vi "PhidgetClose.vi"(8 "error in":errorcluster, 11 "Device In":i32) -> (0 "error out":errorcluster)   [LabVIEW 2013]
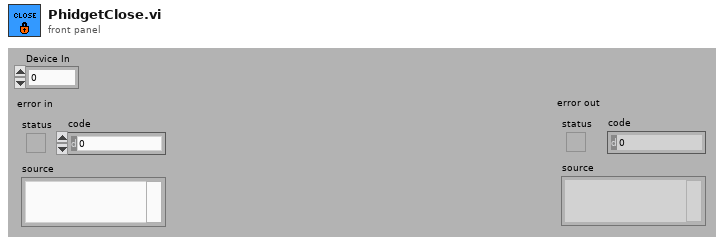
[diagram p1: front panel]
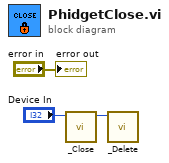
[diagram p0: block diagram]
diagram:
  n1 = call "_Close.vi"("Device In"="Device In") -> ("Device Out"=w1:i32)  [unwired: 9 in, 1 out]
  n2 = call "_Delete.vi"("Device In"=w1) -> ()  [unwired: 10 in, 1 out]
  "error out" <- "error in"
